vi "Simple TCP - Server - Copy 3.vi"() -> ()   [LabVIEW 2021]
doc: "Demonstrates how to set up a basic TCP connection, send data to the specified port once a connection has been established, and terminate the connection once the data has been sent. This VI is designed to stop if the TCP connection is terminated. The data sent in this example is an array of random numbers."
panel:
  out "Waveform Graph 10":dbl[](graph)
  in  "loop 1":i32
  in  "Client Closed":string="The client VI closed the connection."
  in  "Stop":bool
  # "Overview: Demonstrates the use of the TCP functions to initialize a TCP server that can send data to a client VI.\nInstructions:\n1. Run the VI.\n2. Open Simple TCP - Client.vi and follow the instructions on its front panel. Note that if you wait longer than 30 seconds to do this after running this VI, it will time out.\n3. Click Stop to stop the VI. Note that if you stop the client VI, this VI will stop automatically."
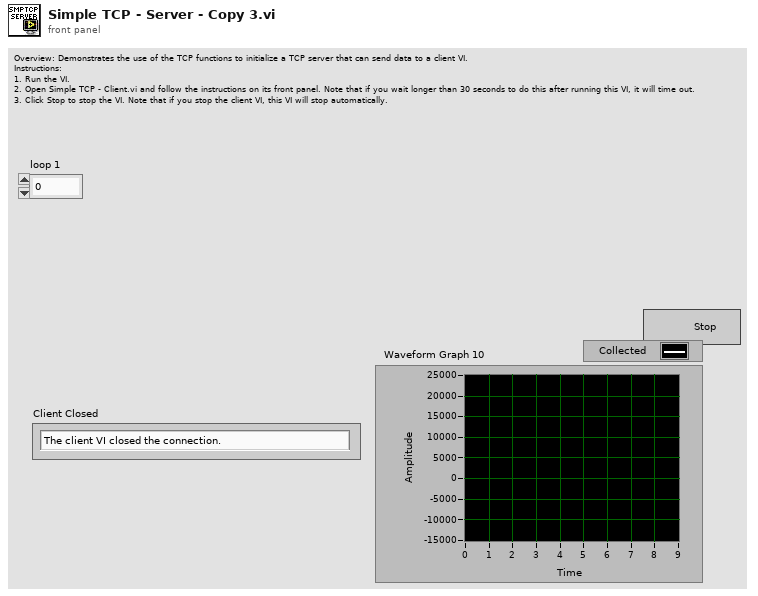
[diagram p1: front panel]
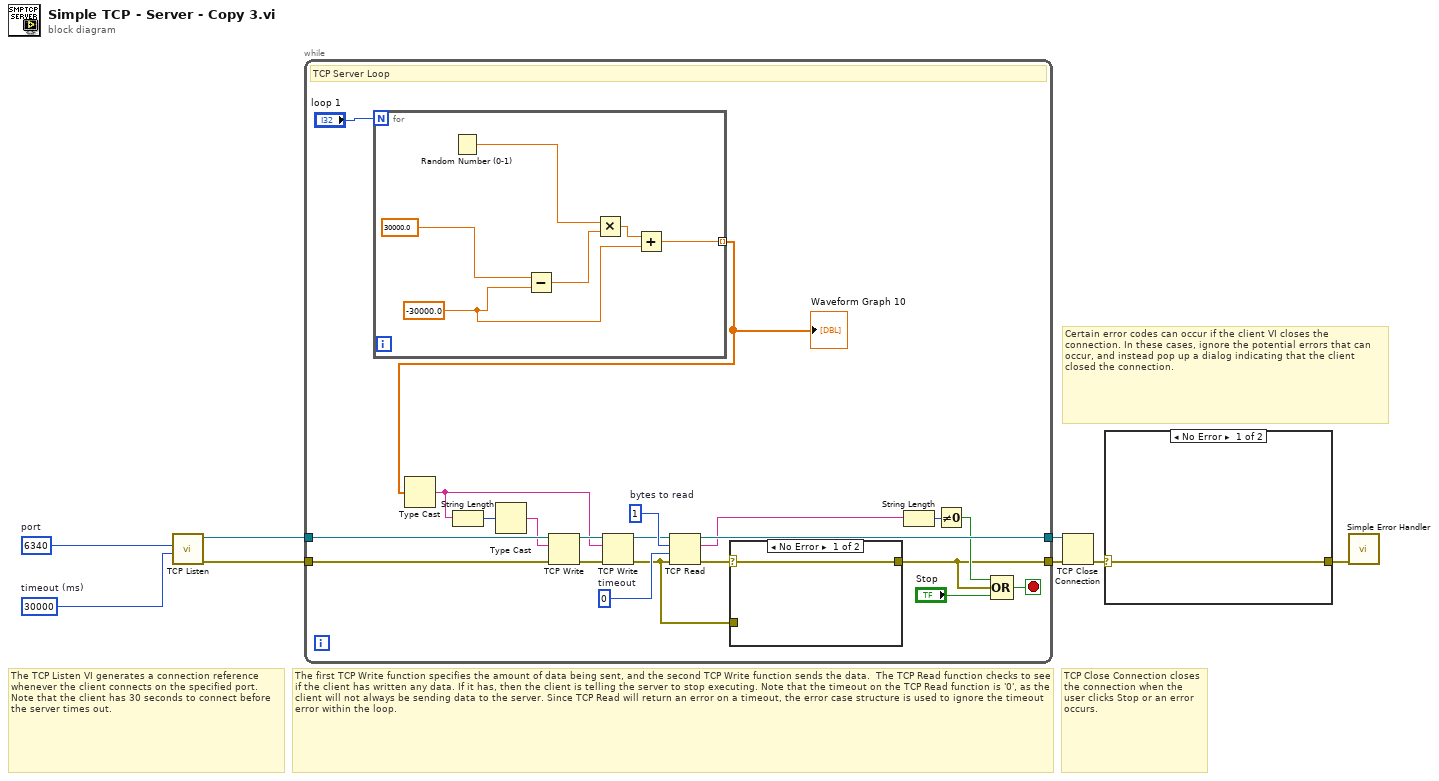
[diagram p0: block diagram]
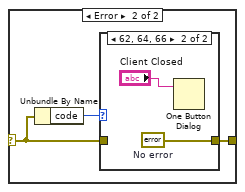
[diagram p2: hidden frame]
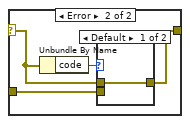
[diagram p4: hidden frame]
diagram:
  w1 = u16 6340  # port
  w2 = 30000  # timeout (ms)
  # "TCP Close Connection closes the connection when the user clicks Stop or an error occurs."
  # "The TCP Listen VI generates a connection reference whenever the client connects on the specified port. Note that the client has 30 seconds to connect before the server times out."
  # "Certain error codes can occur if the client VI closes the connection. In these cases, ignore the potential errors that can occur, and instead pop up a dialog indicating that the client closed the connection."
  # "The first TCP Write function specifies the amount of data being sent, and the second TCP Write function sends the data.  The TCP Read function checks to see if the client has written any data. If it has, then the client is telling the server to stop executing. Note that the timeout on the TCP Read function is '0', as the client will not always be sending data to the server. Since TCP Read will return an error on a timeout, the error case structure is used to ignore the timeout error within the loop."
  n1 = call <vilib>:"TCP Listen.vi"("timeout ms (wait forever: -1)"=w2, "port"=w1) -> ("error out"=w3:errorcluster, "connection ID"=w4:refnum<k5>)  [unwired: 5 in, 3 out]
  n2 = while {
    tunnel: [w12] -> w7
    tunnel: [w18] -> w8
    tunnel: w4 -> [w29]
    tunnel: w3 -> [w22]
    stop <- w23 stop-if-true
    w17 = 0  # timeout
    w20 = 1  # bytes to read
    # "TCP Server Loop"
    n3 = for {
      N: "loop 1" -> [_]
      tunnel: [w30] -> w9 mode=indexing
      w32 = -30000.0 ("y")
      n4 = Random Number (0-1)() -> (number: 0 to 1=w31:dbl)
      n5 = Subtract(x=30000.0, y=w32) -> (x-y=w35:dbl)
      n6 = Multiply(x=w31, y=w35) -> (x*y=w34:dbl)
      n7 = Add(x=w34, y=w32) -> (x+y=w30:dbl)
    }
    "Waveform Graph 10" <- w9
    n8 = Type Cast(x=w9) -> (*(type *) &x=w24:string)  [unwired: 1 out]
    n9 = String Length(string=w24) -> (length=w26:i32)
    n10 = Type Cast(x=w26) -> (*(type *) &x=w25:string)  [unwired: 1 out]
    n11 = TCP Write(connection ID=w29, data in=w25, error in (no error)=w22) -> (connection ID out=w28:refnum<k5>, error out=w27:errorcluster)  [unwired: 2 out]
    n12 = TCP Write(connection ID=w28, data in=w24, error in (no error)=w27) -> (connection ID out=w19:refnum<k5>, error out=w11:errorcluster)  [unwired: 2 out]
    n13 = TCP Read(connection ID=w19, bytes to read=w20, error in (no error)=w11, 9:w17) -> (connection ID out=w18:refnum<k5>, data out=w15:string, error out=w13:errorcluster)  [unwired: 1 out]
    n14 = case shown="No Error" w13 {
      selector: w13 -> [w36 w39]
      tunnel: [w36 w37] -> w12
      tunnel: w11 -> [_ w38]
      frame No Error {
      }
      frame Error {
        n15 = Unbundle By Name(w39) -> ("code"=w40:i32)
        n16 = case shown="Default" w40 {
          tunnel: w39 -> [w41 _]
          tunnel: w38 -> [_ w42]
          tunnel: [w41 w42] -> w37
          frame Default {
          }
          frame 56 {
          }
        }
      }
    }
    n17 = String Length(string=w15) -> (length=w16:i32)
    n18 = Not Equal To 0?(x=w16) -> (x != 0?=w14:bool)
    n19 = Compound Arithmetic op=OR(w14, w12, "Stop") -> (w23:bool)
  }
  n20 = TCP Close Connection(connection ID=w8, error in (no error)=w7) -> (error out=w6:errorcluster)  [unwired: 2 out]
  n21 = case shown="No Error" w6 {
    selector: w6 -> [w43 w45]
    tunnel: [w43 w44] -> w5
    frame No Error {
    }
    frame Error {
      n22 = Unbundle By Name(w45) -> ("code"=w46:i32)
      n23 = case shown="62, 64, 66" w46 {
        tunnel: w45 -> [w47 _]
        tunnel: [w47 w49] -> w44
        frame Default {
        }
        frame 62, 64, 66 {
          w49 = errorcluster {"status"=FALSE, "code"=0, "source"=""}  # No error
          n24 = One Button Dialog(message="Client Closed") -> ()  [unwired: 1 in, 1 out]
        }
      }
    }
  }
  n25 = call <vilib>:"Simple Error Handler.vi"("error in (no error)"=w5) -> ()  [unwired: 1 in, 8 out]
